vi "Can Accept Input.vi"(10 "Input Type":variant, 11 "Dest Type":variant) -> (2 "Can Accept?":bool, 3 "Coercion Needed?":bool)   [LabVIEW 2020, in "FlexBlock.xnode"]
uses:
  FlexBlock.xnode
  <vilib>/Utility/Data Type/NI_Data Type.lvlib
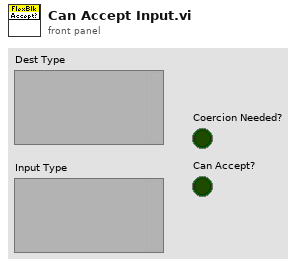
[diagram p1: front panel]
types:
  T1 = typedef "NI_Data Type.lvlib/Data Type.ctl" = enum8{"Invalid Type", "Void", "I8", "I16", "I32", "I64", "U8", "U16", "U32", "U64", "Single Float", "Double Float", "Extended Float", "Single Complex", "Double Complex", "Extended Complex", "Enum U8", "Enum U16", "Enum U32", "Enum U64", "Single Float With Unit", "Double Float With Unit", "Extended Float With Unit", "Single Complex with Unit", "Double Complex with Unit", "Extended Complex with Unit", "Boolean", "String", "Path", "Picture", "Tag", "Array", "Cluster", "Variant", "LV Variant", "Waveform", "Timestamp", "Digital Waveform", "Digital Data", "ExpressData", "Refnum", "External Data", "VI", "Poly VI", "LabVIEW Class Instance", "Fixed Point", "Set Collection", "Map Collection"}
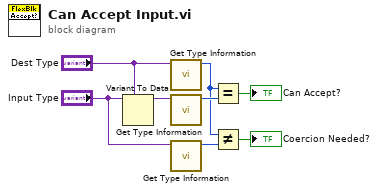
[diagram p0: block diagram]
diagram:
  n1 = Variant To Data(type="Dest Type", Variant="Input Type") -> (data=w8:variant)  [unwired: 1 in, 1 out]
  n2 = call <vilib>:"Get Type Information.vi"("variant"="Dest Type") -> ("type"=w2:T1)  [unwired: 6 in, 4 out]
  n3 = call <vilib>:"Get Type Information.vi"("variant"=w8) -> ("type"=w7:T1)  [unwired: 6 in, 4 out]
  n4 = call <vilib>:"Get Type Information.vi"("variant"="Input Type") -> ("type"=w3:T1)  [unwired: 6 in, 4 out]
  n5 = Equal?(x=w2, y=w7) -> (x = y?=→"Can Accept?":bool)
  n6 = Not Equal?(x=w2, y=w3) -> (x != y?=→"Coercion Needed?":bool)
